vi "which_extension.vi"(11 "Image path":path) -> (3 "image data":T1)   [LabVIEW 2023]
doc: "Returns picture extension"
uses:
  <vilib>/picture/picture.llb/imagedata.ctl
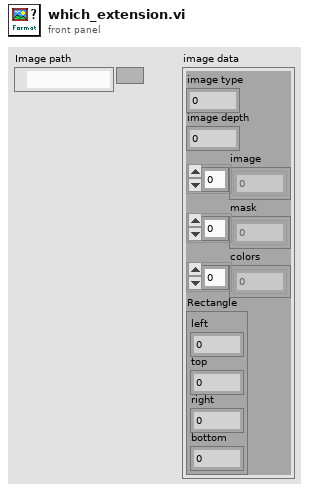
[diagram p1: front panel]
types:
  T1 = typedef "imagedata.ctl" = cluster{"image type":i32, "image depth":i32, "image":u8[], "mask":u8[], "colors":u32[], "Rectangle":cluster{"left":i16, "top":i16, "right":i16, "bottom":i16}}
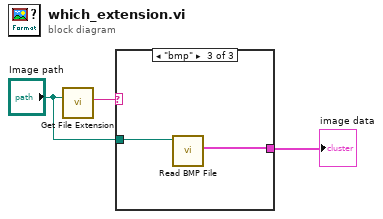
[diagram p0: block diagram]
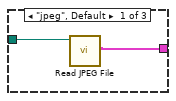
[diagram p2: hidden frame]
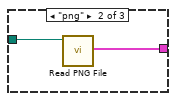
[diagram p3: hidden frame]
diagram:
  n1 = call <vilib>:"Get File Extension.vi"("file"="Image path") -> ("lowercase file extension"=w1:string)  [unwired: 6 in, 4 out]
  n2 = case shown="\"bmp\"" w1 {
    tunnel: "Image path" -> [w5 w7 w9]
    tunnel: [w4 w6 w8] -> w3
    frame "jpeg", Default {
      n3 = call <vilib>:"Read JPEG File.vi"("path to JPEG file"=w5) -> ("image data"=w4:T1)  [unwired: 8 in, 2 out]
    }
    frame "png" {
      n4 = call <vilib>:"Read PNG File.vi"("path to PNG file"=w7) -> ("image data"=w6:T1)  [unwired: 8 in, 2 out]
    }
    frame "bmp" {
      n5 = call <vilib>:"Read BMP File.vi"("path to BMP file"=w9) -> ("image data"=w8:T1)  [unwired: 8 in, 2 out]
    }
  }
  "image data" <- w3
